vi "Load Part Config Data.vi"(11 "All Part Info":T1=[{"Type Name"="", "Type Signal Names"=["1"], "# Signals"=1, "# Parts"=0, "Part Info"=[]}]) -> (3 "All Part Info Out":T3(array[cluster]))   [LabVIEW 2019]
uses:
  Type Defs and Controls/Part Info.ctl
  Type Defs and Controls/All Part Info.ctl
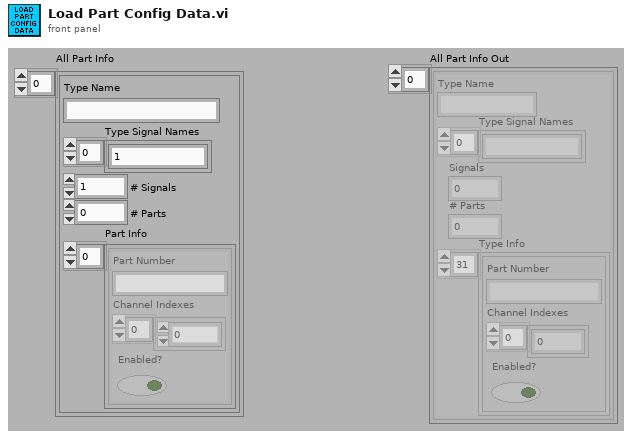
[diagram p1: front panel]
types:
  T1 = typedef "All Part Info.ctl" = cluster{"Type Name":string, "Type Signal Names":string[], "# Signals":i32, "# Parts":i32, "Part Info":T2[]}[]
  T2 = typedef "Part Info.ctl" = cluster{"Part Number":string, "Channel Indexes":u16[], "Enabled?":bool}
  T3 = cluster{"Type Name":string, "Type Signal Names":string[], "Signals":i32, "# Parts":i32, "Type Info":T2[]}[]
  T4 = cluster{"Type Name":string, "Type Signal Names":string[], "# Signals":i32, "# Parts":i32, "Part Info":T2[]}
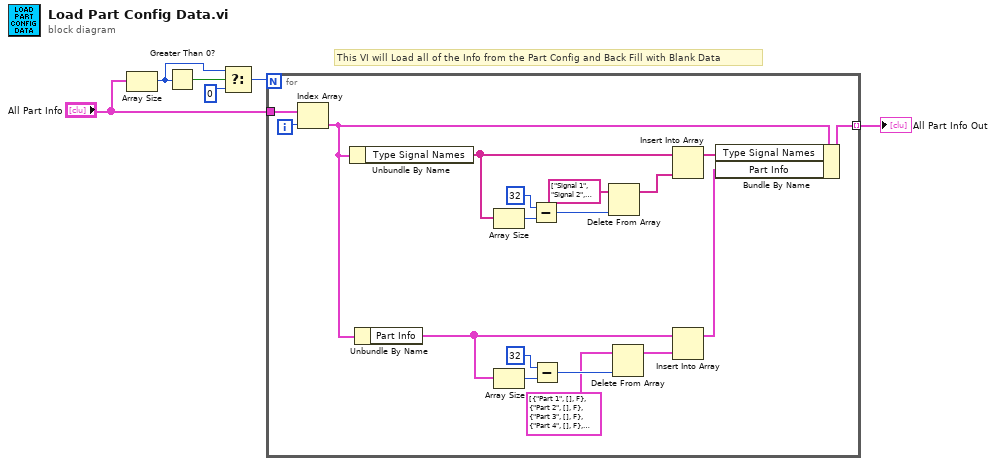
[diagram p0: block diagram]
diagram:
  # "This VI will Load all of the Info from the Part Config and Back Fill with Blank Data"
  n1 = Array Size(array="All Part Info") -> (size(s)=w2:i32)
  n2 = Greater Than 0?(x=w2) -> (x > 0?=w4:bool)
  n3 = Select(t=w2, s=w4, f=0) -> (s? t:f=w1:i32)
  n4 = for {
    N: w1 -> [_]
    tunnel: "All Part Info" -> [w19]
    tunnel: [w20] -> w6 mode=indexing
    i -> [w18]
    n5 = Index Array(array=w19, index=w18) -> (element=w17:T4)
    n6 = Unbundle By Name(w17) -> ("Type Signal Names"=w22:string[])
    n7 = Unbundle By Name(w17) -> ("Part Info"=w14:T2[])
    n8 = Array Size(array=w22) -> (size(s)=w24:i32)
    n9 = Array Size(array=w14) -> (size(s)=w15:i32)
    n10 = Subtract(x=32, y=w24) -> (x-y=w11:i32)
    n11 = Subtract(x=32, y=w15) -> (x-y=w9:i32)
    n12 = Delete From Array(array=string[] ["Signal 1", "Signal 2", "Signal 3", "Signal 4", "Signal 5", "Signal 6", "Signal 7", "Signal 8", "Signal 9", "Signal 10", "Signal 11", "Signal 12", "Signal 13", "Signal 14", "Signal 15", "Signal 16", "Signal 17", "Signal 18", "Signal 19", "Signal 20", "Signal 21", "Signal 22", "Signal 23", "Signal 24", "Signal 25", "Signal 26", "Signal 27", "Signal 28", "Signal 29", "Signal 30", "Signal 31", "Signal 32"] ("Array"), index=w11) -> (array with subset deleted=w10:string[])  [unwired: 1 in, 1 out]
    n13 = Delete From Array(array=T2[] [{"Part Number"="Part 1", "Channel Indexes"=[], "Enabled?"=FALSE}, {"Part Number"="Part 2", "Channel Indexes"=[], "Enabled?"=FALSE}, {"Part Number"="Part 3", "Channel Indexes"=[], "Enabled?"=FALSE}, {"Part Number"="Part 4", "Channel Indexes"=[], "Enabled?"=FALSE}, {"Part Number"="Part 5", "Channel Indexes"=[], "Enabled?"=FALSE}, {"Part Number"="Part 6", "Channel Indexes"=[], "Enabled?"=FALSE}, {"Part Number"="Part 7", "Channel Indexes"=[], "Enabled?"=FALSE}, {"Part Number"="Part 8", "Channel Indexes"=[], "Enabled?"=FALSE}, {"Part Number"="Part 9", "Channel Indexes"=[], "Enabled?"=FALSE}, {"Part Number"="Part 10", "Channel Indexes"=[], "Enabled?"=FALSE}, {"Part Number"="Part 11", "Channel Indexes"=[], "Enabled?"=FALSE}, {"Part Number"="Part 12", "Channel Indexes"=[], "Enabled?"=FALSE}, {"Part Number"="Part 13", "Channel Indexes"=[], "Enabled?"=FALSE}, {"Part Number"="Part 14", "Channel Indexes"=[], "Enabled?"=FALSE}, {"Part Number"="Part 15", "Channel Indexes"=[], "Enabled?"=FALSE}, {"Part Number"="Part 16", "Channel Indexes"=[], "Enabled?"=FALSE}, {"Part Number"="Part 17", "Channel Indexes"=[], "Enabled?"=FALSE}, {"Part Number"="Part 18", "Channel Indexes"=[], "Enabled?"=FALSE}, {"Part Number"="Part 19", "Channel Indexes"=[], "Enabled?"=FALSE}, {"Part Number"="Part 20", "Channel Indexes"=[], "Enabled?"=FALSE}, {"Part Number"="Part 21", "Channel Indexes"=[], "Enabled?"=FALSE}, {"Part Number"="Part 22", "Channel Indexes"=[], "Enabled?"=FALSE}, {"Part Number"="Part 23", "Channel Indexes"=[], "Enabled?"=FALSE}, {"Part Number"="Part 24", "Channel Indexes"=[], "Enabled?"=FALSE}, {"Part Number"="Part 25", "Channel Indexes"=[], "Enabled?"=FALSE}, {"Part Number"="Part 26", "Channel Indexes"=[], "Enabled?"=FALSE}, {"Part Number"="Part 27", "Channel Indexes"=[], "Enabled?"=FALSE}, {"Part Number"="Part 28", "Channel Indexes"=[], "Enabled?"=FALSE}, {"Part Number"="Part 29", "Channel Indexes"=[], "Enabled?"=FALSE}, {"Part Number"="Part 30", "Channel Indexes"=[], "Enabled?"=FALSE}, {"Part Number"="Part 31", "Channel Indexes"=[], "Enabled?"=FALSE}, {"Part Number"="Part 32", "Channel Indexes"=[], "Enabled?"=FALSE}] ("Array"), index=w9) -> (array with subset deleted=w8:T2[])  [unwired: 1 in, 1 out]
    n14 = Insert Into Array(array=w22, new element=w10) -> (w21:string[])  [unwired: 1 in]
    n15 = Insert Into Array(array=w14, new element=w8) -> (w13:T2[])  [unwired: 1 in]
    n16 = Bundle By Name(cluster=w17, "Type Signal Names"=w21, "Part Info"=w13) -> (w20:T4)
  }
  "All Part Info Out" <- w6
